vi "LabVIEWBasicPythonCall.vi"() -> ()   [LabVIEW 2021]
doc: "Basic example of calling Python function in LabVIEW"
panel:
  in  "c":dbl=2.0
  in  "b":dbl=2.0
  in  "a":dbl=2.0
  out "DELTA":dbl format="%.2f"
  out "Error Out":errorcluster
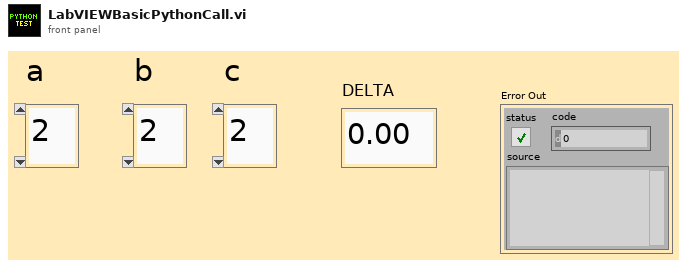
[diagram p1: front panel]
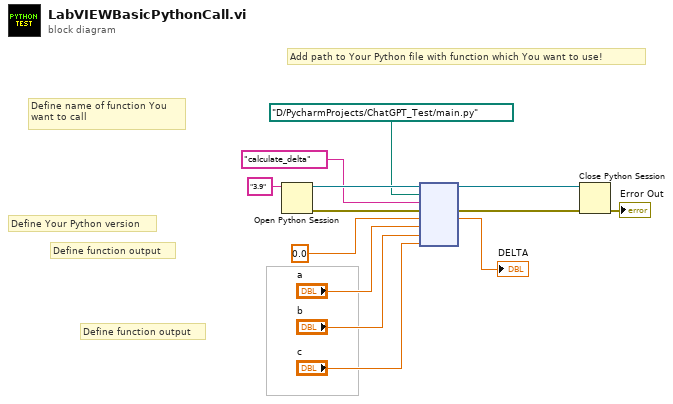
[diagram p0: block diagram]
diagram:
  # "Define function output"
  # "Define function output"
  # "Define name of function You\nwant to call"
  # "Define Your Python version"
  # "Add path to Your Python file with function which You want to use!"
  n1 = Open Python Session(python version="3.9" ("Python version")) -> (session out=w12:refnum<k35>, error out=w4:errorcluster)  [unwired: 2 in]
  n2 = node(w12, path "D:/PycharmProjects/ChatGPT_Test/main.py" ("module path"), "calculate_delta" ("function name"), w4, 0.0 ("out"), "a", "b", "c") -> (w9:refnum<k35>, w8:errorcluster, →"DELTA":dbl)  [unwired: 3 in, 2 out]
  n3 = Close Python Session(session in=w9, error in=w8) -> (11:→"Error Out":errorcluster)
